vi "UpdateAutoLog.vi"(8 "error in":errorcluster, 10 "Log Array":string[](array[string])) -> (0 "error out":errorcluster)   [LabVIEW 2015]
uses:
  <vilib>/Rock Robotics/Network Tables/NT Write String.vi
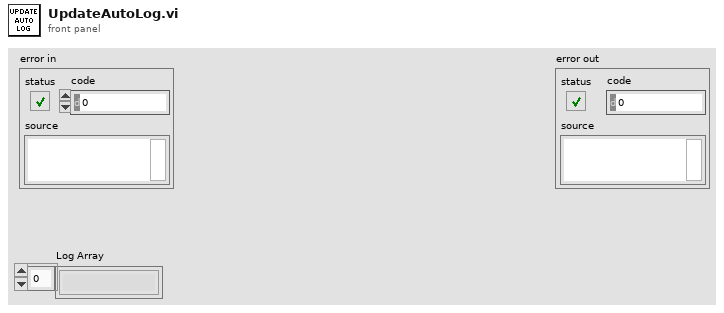
[diagram p1: front panel]
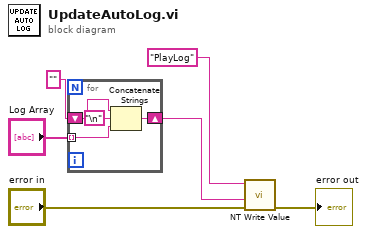
[diagram p0: block diagram]
diagram:
  n1 = for {
    tunnel: "Log Array" -> [w10] mode=indexing
    shift-right: [w9] -> w1
    shift-left: "" -> [w8]
    n2 = Concatenate Strings(w8, "\n", w10) -> (w9:string)
  }
  n3 = call-poly <vilib>:"NT Write Value.vi"("error in"="error in", "String"=w1, "Name"="PlayLog") -> ("error out"=→"error out":errorcluster)  [unwired: 8 in]
